vi "Agilent34410A Set Range.vi"(8 "error in (no error)":errorcluster, 9 "Range String":string, 10 "DMM Function":T1, 11 "VISA Rsrc":refnum<visa-resource-name>="SR530") -> (0 "error out":errorcluster, 3 "VISA Rsrc Out":refnum<visa-resource-name>="GPIB0::12::INSTR", 4 "ChaineCom":string caption="Chaîne de commande")   [LabVIEW 2019]
uses:
  <userlib>/Agilent34410A/Agilent34410A DMM_Func.ctl
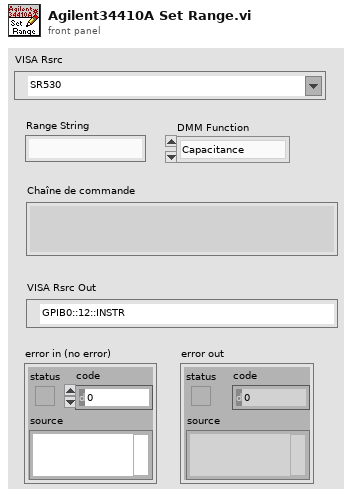
[diagram p1: front panel]
types:
  T1 = typedef "Agilent34410A DMM_Func.ctl" = enum16{"Capacitance", "Continuity", "Current AC", "Current", "Diode", "Frequency", "4W Resistance", "Period", "Resistance", "Temperature", "Voltage AC", "Voltage"}
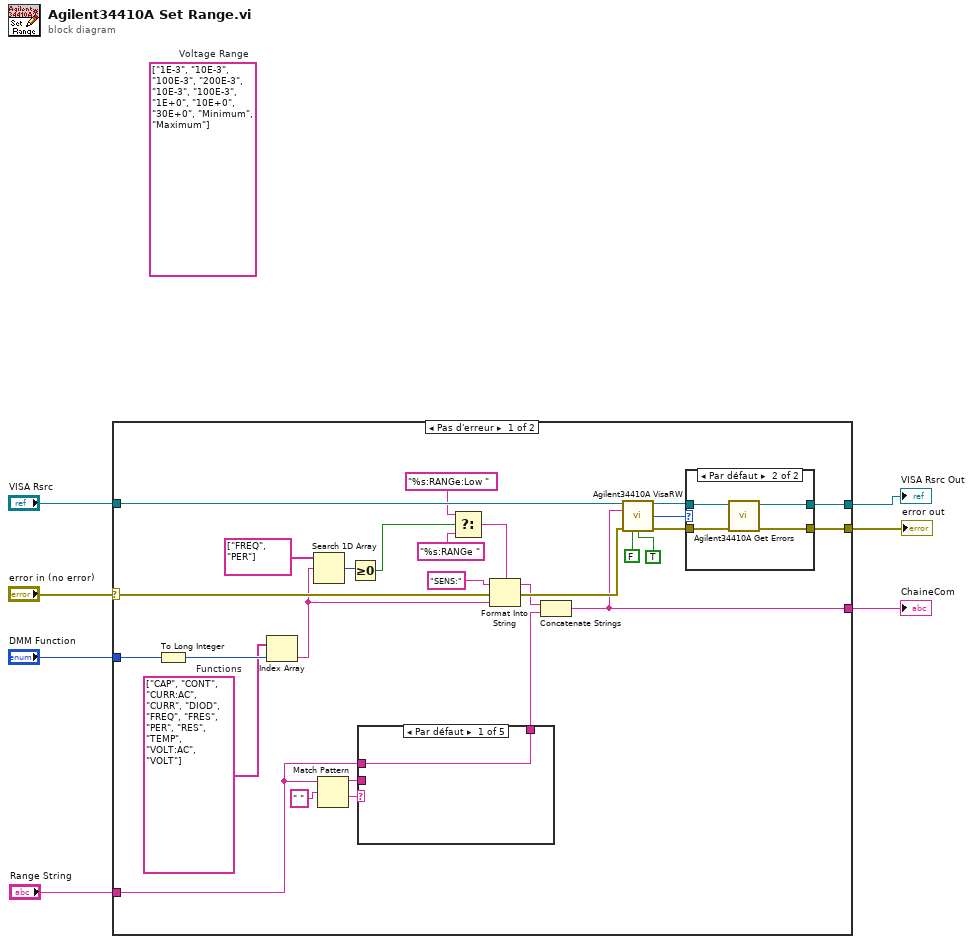
[diagram p0: block diagram]
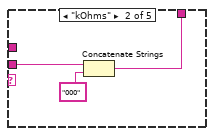
[diagram p2: hidden frame]
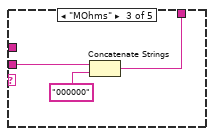
[diagram p3: hidden frame]
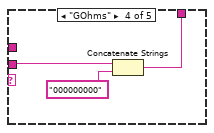
[diagram p4: hidden frame]
diagram:
  (unwired) string[] ["1E-3", "10E-3", "100E-3", "200E-3", "10E-3", "100E-3", "1E+0", "10E+0", "30E+0", "Minimum", "Maximum"]  # Voltage Range
  n1 = case shown="Pas d'erreur" "error in (no error)" {
    selector: "error in (no error)" -> [w32 w53]
    tunnel: "VISA Rsrc" -> [w35 w54]
    tunnel: [w25 w53] -> w5
    tunnel: [w26 w54] -> w4
    tunnel: [w21 _] -> w3
    tunnel: "Range String" -> [w9 _]
    tunnel: "DMM Function" -> [w24 _]
    frame No Error {
      w19 = string[] ["CAP", "CONT", "CURR:AC", "CURR", "DIOD", "FREQ", "FRES", "PER", "RES", "TEMP", "VOLT:AC", "VOLT"]  # Functions
      n2 = To Long Integer(number=w24) -> (32bit integer=w23:i32)
      n3 = Index Array(array=w19, index=w23) -> (element=w18:string)
      n4 = Search 1D Array(1D array=string[] ["FREQ", "PER"], element=w18) -> (index of element=w17:i32)  [unwired: 1 in]
      n5 = Match Pattern(string=w9, regular expression=" " ("expression régulière")) -> (before substring=w8:string, after substring=w11:string)  [unwired: 1 in, 2 out]
      n6 = Greater Or Equal To 0?(x=w17) -> (x >= 0?=w16:bool)
      n7 = case shown="Par défaut" w11 {
        tunnel: [w36 w37 w40 w43 w46] -> w10
        tunnel: w9 -> [w36 _ _ _ _]
        tunnel: w8 -> [_ w39 w41 w44 w46]
        frame Default {
        }
        frame "kOhms" {
          n8 = Concatenate Strings(w39, "000" ("chaîne")) -> (w37:string)
        }
        frame "MOhms" {
          n9 = Concatenate Strings(w41, "000000" ("chaîne")) -> (w40:string)
        }
        frame "GOhms" {
          n10 = Concatenate Strings(w44, "000000000" ("chaîne")) -> (w43:string)
        }
        frame "Ohms" {
        }
      }
      n11 = Select(t="%s:RANGe:Low " ("string (\"\")"), s=w16, f="%s:RANGe " ("string (\"\")")) -> (s? t:f=w13:string)
      n12 = Format Into String(format string=w13, initial string="SENS:" ("string (\"\")"), error in=w32, w18) -> (resulting string=w22:string, error out=w31:errorcluster)
      n13 = Concatenate Strings(w22, w10) -> (w21:string)
      n14 = call <userlib>:"Agilent34410A VisaRW.vi"("VISA Rsrc"=w35, "ChaineCom"=w21, "error in (no error)"=w31, "Lecture?(T)"=FALSE, "Poll?(F)"=TRUE) -> ("VISA Rsrc Out"=w27:refnum<visa-resource-name>, "octet d'état"=w28:u16, "error out"=w29:errorcluster)  [unwired: 6 in, 2 out]
      n15 = case shown="Par défaut" w28 {
        tunnel: w27 -> [w48 w52]
        tunnel: w29 -> [w47 w51]
        tunnel: [w47 w50] -> w25
        tunnel: [w48 w49] -> w26
        frame 0 {
        }
        frame Default {
          n16 = call <userlib>:"Agilent34410A Get Errors.vi"("error in (no error)"=w51, "VISA Rsrc"=w52) -> ("error out"=w50:errorcluster, "VISA Rsrc Out"=w49:refnum<visa-resource-name>)  [unwired: 7 in, 1 out]
        }
      }
    }
    frame Error {
    }
  }
  "error out" <- w5
  "VISA Rsrc Out" <- w4
  "ChaineCom" <- w3
